vi "Configure Modulation Waveform (Swept-Sine).vi"(6 "Sweep Trigger (1: Immediate)":u16(ring)=1 items=["Bus", "Immediate", "External", "Key"], 7 "Modulation Path (1)":u16(ring)=1 items=["1"=1, "2"=2], 8 "error in (no error)":errorcluster, 9 "Sweep Rate (400 Hz)":dbl=400.0, 10 "Modulation Type (0: Amplitude Modulation)":u16(ring) items=["Amplitude Modulation", "Frequency Modulation", "Phase Modulation", "Low Frequency Output"], 11 "VISA resource name":refnum<visa-resource-name>) -> (0 "error out":errorcluster, 3 "VISA resource name out":refnum<visa-resource-name>)   [LabVIEW 2011, in "Agilent PSG MXG Series.lvlib"]
doc: "Configures the sweep rate and trigger source for the swept-sine waveform.\n\n<B>Notes:</B>\n(1) This VI is <B>NOT</B> valid in E8247C, N5181A, N5182A, N5183A.\n\n(2) For E8257D, E8267D, this VI is valid only when the instrument installs <B>Option UNT</B> (AM, FM, phase modulation, and LF output)."
uses:
  Agilent PSG MXG Series.lvlib
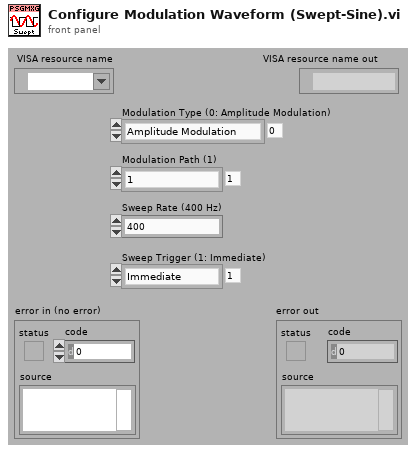
[diagram p1: front panel]
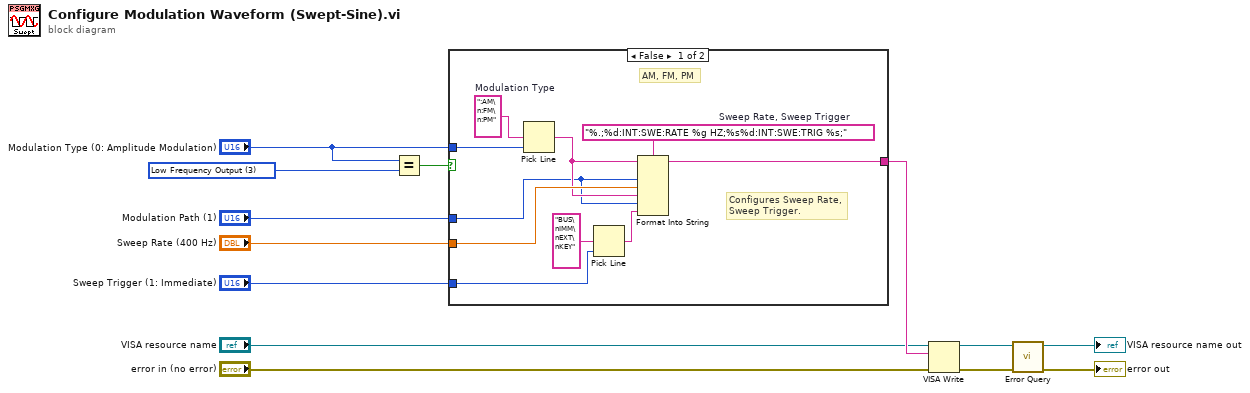
[diagram p0: block diagram]
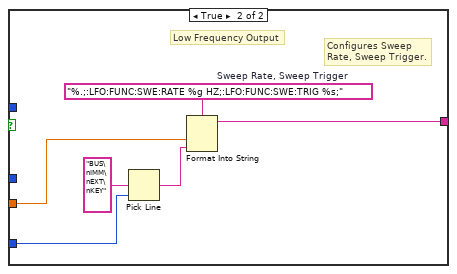
[diagram p2: hidden frame]
diagram:
  w9 = u16 3 items=["Amplitude Modulation", "Frequency Modulation", "Phase Modulation", "Low Frequency Output"] ("Modulation Type (0: Amplitude Modulation)")
  n1 = Equal?(x="Modulation Type (0: Amplitude Modulation)", y=w9) -> (x = y?=w13:bool)
  n2 = case shown="False" w13 {
    tunnel: "Modulation Type (0: Amplitude Modulation)" -> [w22 _]
    tunnel: "Modulation Path (1)" -> [w17 _]
    tunnel: "Sweep Rate (400 Hz)" -> [w21 w28]
    tunnel: [w20 w27] -> w12
    tunnel: "Sweep Trigger (1: Immediate)" -> [w15 w24]
    frame False {
      w19 = "%.;%d:INT:SWE:RATE %g HZ;%s%d:INT:SWE:TRIG %s;"  # Sweep Rate, Sweep Trigger
      w23 = ":AM\n:FM\n:PM"  # Modulation Type
      # "Configures Sweep Rate,\nSweep Trigger."
      # "AM, FM, PM"
      n3 = Pick Line(multi-line string=w23, line index=w22) -> (output string=w18:string)  [unwired: 1 in]
      n4 = Pick Line(multi-line string="BUS\nIMM\nEXT\nKEY", line index=w15) -> (output string=w14:string)  [unwired: 1 in]
      n5 = Format Into String(format string=w19, initial string=w18, w17, w21, w18, w17, w14) -> (resulting string=w20:string)  [unwired: 1 in, 1 out]
    }
    frame True {
      w29 = "%.;:LFO:FUNC:SWE:RATE %g HZ;:LFO:FUNC:SWE:TRIG %s;"  # Sweep Rate, Sweep Trigger
      # "Configures Sweep\nRate, Sweep Trigger."
      # "Low Frequency Output"
      n6 = Pick Line(multi-line string="BUS\nIMM\nEXT\nKEY", line index=w24) -> (output string=w26:string)  [unwired: 1 in]
      n7 = Format Into String(format string=w29, w28, w26) -> (resulting string=w27:string)  [unwired: 2 in, 1 out]
    }
  }
  n8 = VISA Write(VISA resource name="VISA resource name", write buffer=w12, error in (no error)="error in (no error)") -> (VISA resource name out=w11:refnum<visa-resource-name>, error out=w10:errorcluster)  [unwired: 1 out]
  n9 = call "Error Query.vi"("error in (no error)"=w10, "VISA resource name"=w11) -> ("error out"=→"error out":errorcluster, "VISA resource name out"=→"VISA resource name out":refnum<visa-resource-name>)  [unwired: 6 in, 2 out]
